vi "CaseStruct.vi"() -> ()   [LabVIEW 2020]
uses:
  <vilib>/ErrorRing/Error Ring.xnode
panel:
  in  "Knob":dbl(knob) scale=0.0..10.0
  in  "String":string
  in  "Boolean":bool
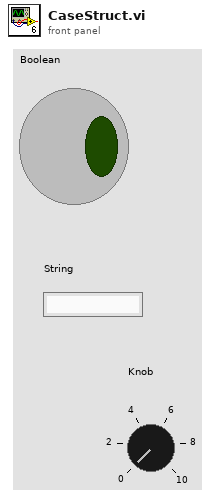
[diagram p1: front panel]
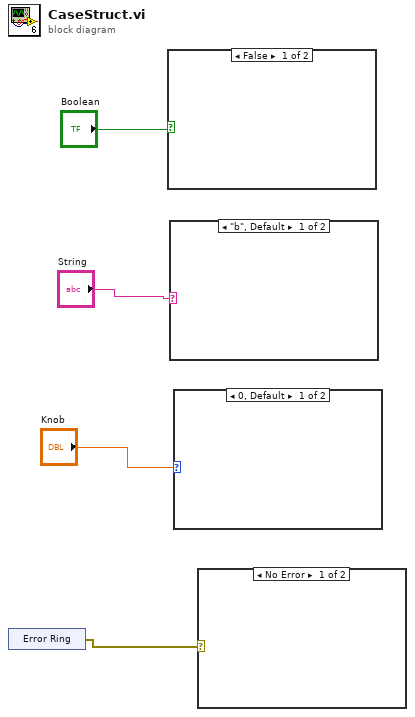
[diagram p0: block diagram]
diagram:
  n1 = xnode "Error Ring"() -> ("error out"=w1:errorcluster)
  n2 = case shown="False" "Boolean" {
    frame False {
    }
    frame True {
    }
  }
  n3 = case shown="\"b\", Default" "String" {
    frame "b", Default {
    }
    frame "a" {
    }
  }
  n4 = case shown="0, Default" "Knob" {
    frame 0, Default {
    }
    frame 8 {
    }
  }
  n5 = case shown="No Error" w1 {
    frame No Error {
    }
    frame Error {
    }
  }
